vi "DataMult.vi"(1 "Divider":i32, 2 "Data IN":dbl[][](array[numeric])) -> (0 "Data OUT":dbl[][](array[numeric]))   [LabVIEW 2012]
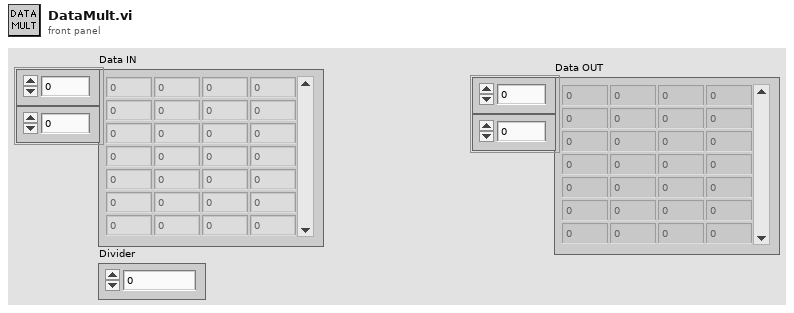
[diagram p1: front panel]
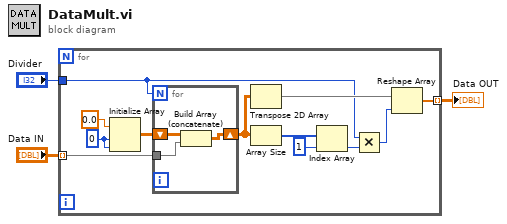
[diagram p0: block diagram]
diagram:
  n1 = for {
    tunnel: "Data IN" -> [w15] mode=indexing
    tunnel: "Divider" -> [w7]
    tunnel: [w4] -> w1 mode=indexing
    w11 = 0 ("dimension size")
    n2 = Initialize Array(0.0 ("element"), w11, w11) -> (w13:dbl[][])
    n3 = for {
      N: w7 -> [_]
      shift-right: [w18] -> w10
      shift-left: w13 -> [w17]
      tunnel: w15 -> [w16]
      n4 = Build Array (concatenate)(w17, w16) -> (w18:dbl[][])
    }
    n5 = Transpose 2D Array(2D array=w10) -> (transposed array=w14:dbl[][])
    n6 = Array Size(array=w10) -> (size(s)=w9:i32[])
    n7 = Index Array(array=w9, index=1) -> (element=w6:i32)
    n8 = Multiply(x=w7, y=w6) -> (x*y=w5:i32)
    n9 = Reshape Array(w14, w5) -> (w4:dbl[])
  }
  "Data OUT" <- w1
